vi "DisplayStriptestData.vi"(5 "Strip Lengths [cm]":dbl[](array[numeric]), 6 "min scale array":i32[](array[numeric]), 7 "max scale array":i32[](array[numeric]), 8 "# probed":i32, 9 "Display Stats?":bool, 10 "Thresholds:":T1={"Current [nA]"=200.0, "Ccoupl Lo [pF/cm]"=20.0, "Ccoupl Hi [pF/cm]"=33.0, "Rbias Lo [MW]"=1.0, "Rbias Hi [MW]"=2.0}, 11 "Region":i32) -> (0 "Defects":i32[][](graph), 1 "Resistance [MW]":cluster{u32, i32, "Array OUT":dbl[]}(graph), 2 "Capacitance [pF]":cluster{u32, i32, "Array OUT":dbl[]}(graph), 3 "Current [nA]":cluster{u32, i32, "Array OUT":dbl[]}(graph), 4 "Strip Quality Data":T2 {"pass Rate in %" format="%.2f"})   [LabVIEW 2018]
panel:
  out "max scale":i32
  out "min scale":i32
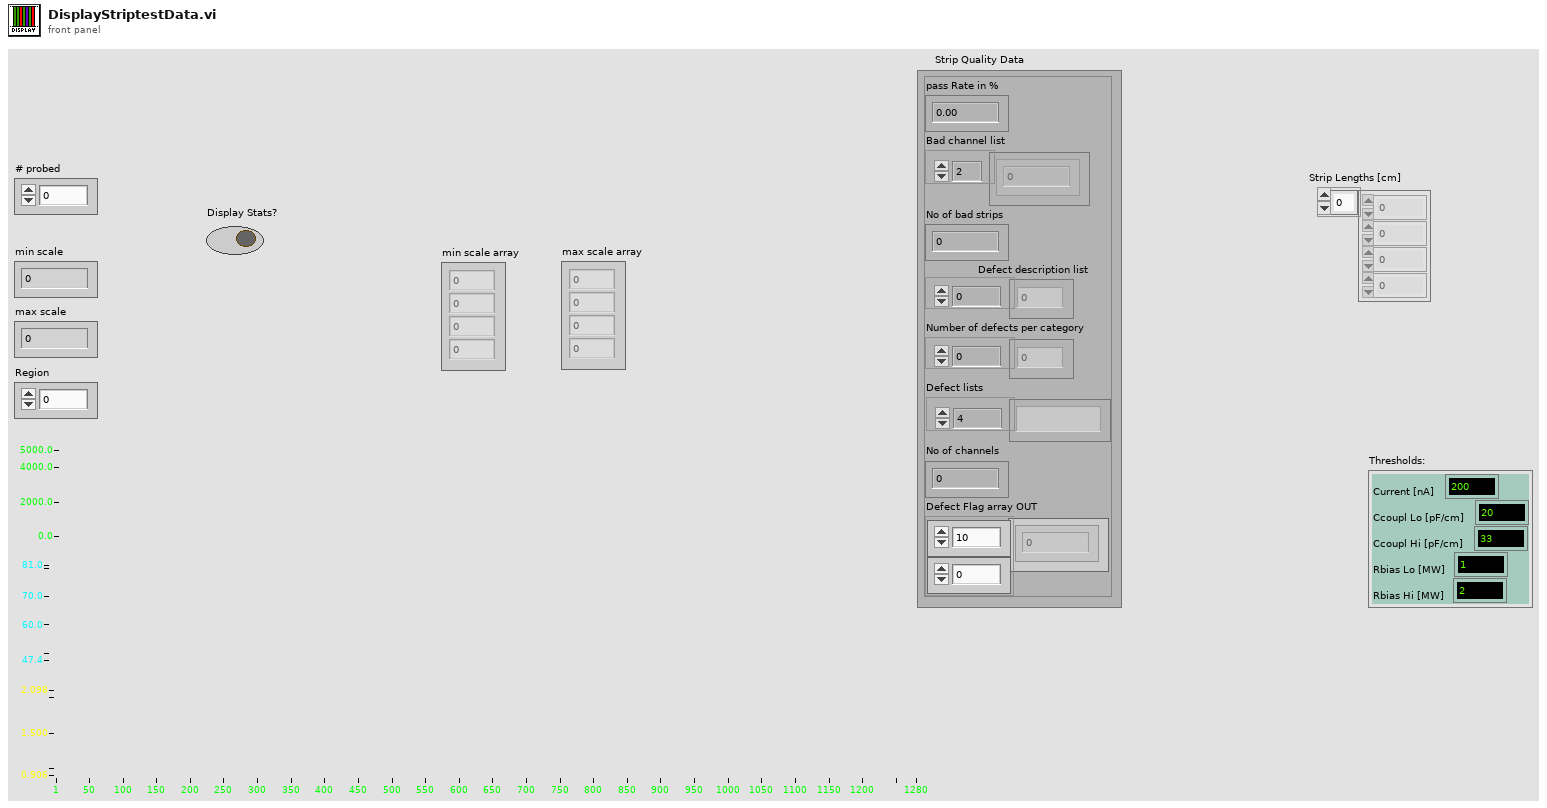
[diagram p1: front panel]
types:
  T1 = cluster{"Current [nA]":dbl, "Ccoupl Lo [pF/cm]":dbl, "Ccoupl Hi [pF/cm]":dbl, "Rbias Lo [MW]":dbl, "Rbias Hi [MW]":dbl}
  T2 = cluster{"pass Rate in %":dbl, "Bad channel list":i32[], "No of bad strips":i32, "Defect description list":i32[], "Number of defects per category":i32[], "Defect lists":string[], "No of channels":i32, "Defect Flag array OUT":i32[][]}
  T3 = enum16{"Reset", "Read Array", "Read Element", "Write Element", "Write Array", "Add Element", "Add Array"}
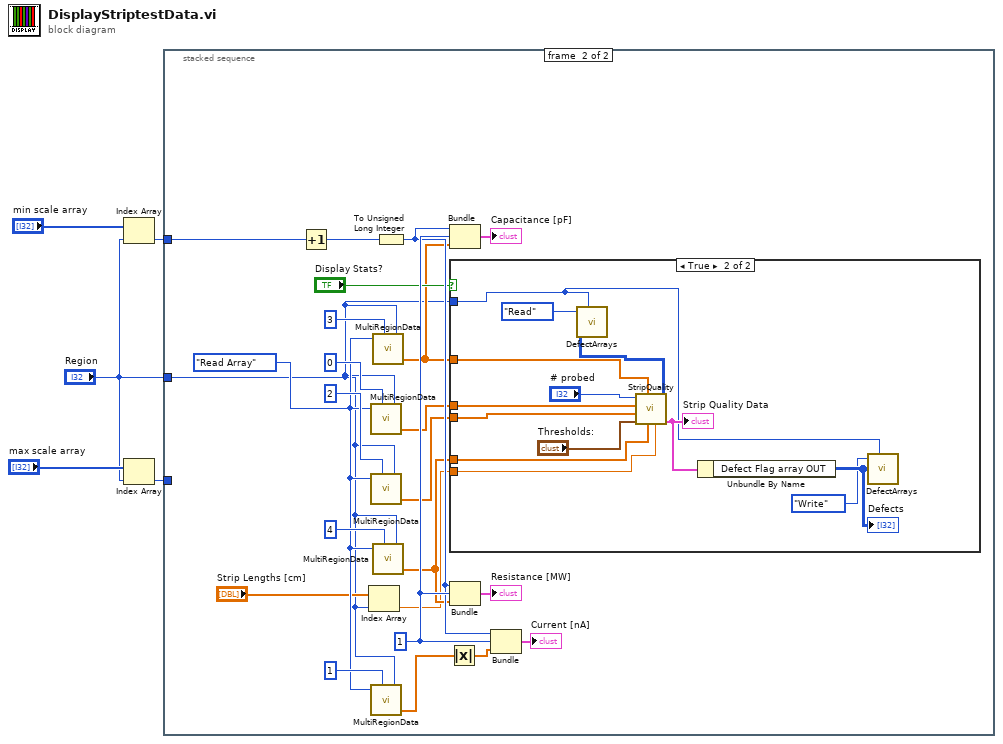
[diagram p0: block diagram]
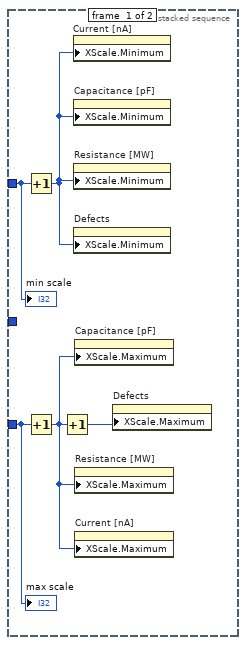
[diagram p2: hidden frame]
diagram:
  n1 = Index Array(array="min scale array", index="Region") -> (element=w4:i32)
  n2 = Index Array(array="max scale array", index="Region") -> (element=w2:i32)
  n3 = stacked-sequence {
    tunnel: w4 -> [w10 w16]
    tunnel: w2 -> [w8 _]
    tunnel: "Region" -> [_ w12]
    frame #0 {
      n4 = Increment(x=w10) -> (x+1=w9:i32)
      n5 = Increment(x=w8) -> (x+1=w7:i32)
      n6 = Increment(x=w7) -> (x+1=w6:i32)
      n7 = property on="Current [nA]" class="WFGraph (strict)"("XScale.Minimum"=w9) -> ()  [unwired: 2 in, 2 out]
      n8 = property on="Capacitance [pF]" class="WFGraph (strict)"("XScale.Minimum"=w9) -> ()  [unwired: 2 in, 2 out]
      n9 = property on="Resistance [MW]" class="WFGraph (strict)"("XScale.Minimum"=w9) -> ()  [unwired: 2 in, 2 out]
      n10 = property on="Defects" class="IntGraph (strict)"("XScale.Minimum"=w9) -> ()  [unwired: 2 in, 2 out]
      n11 = property on="Capacitance [pF]" class="WFGraph (strict)"("XScale.Maximum"=w7) -> ()  [unwired: 2 in, 2 out]
      n12 = property on="Resistance [MW]" class="WFGraph (strict)"("XScale.Maximum"=w7) -> ()  [unwired: 2 in, 2 out]
      n13 = property on="Current [nA]" class="WFGraph (strict)"("XScale.Maximum"=w7) -> ()  [unwired: 2 in, 2 out]
      n14 = property on="Defects" class="IntGraph (strict)"("XScale.Maximum"=w6) -> ()  [unwired: 2 in, 2 out]
      "min scale" <- w10
      "max scale" <- w8
    }
    frame #1 {
      w14 = T3."Read Array" ("Action")
      w28 = 1
      n15 = Increment(x=w16) -> (x+1=w15:i32)
      n16 = Index Array(array="Strip Lengths [cm]", index=w12) -> (element=w11:dbl)
      n17 = call "MultiRegionData.vi"("Action"=w14, "Array No."=0, "Region index"=w12) -> ("Array OUT"=w20:dbl[])  [unwired: 3 in, 1 out]
      n18 = call "MultiRegionData.vi"("Action"=w14, "Array No."=2, "Region index"=w12) -> ("Array OUT"=w17:dbl[])  [unwired: 3 in, 1 out]
      n19 = call "MultiRegionData.vi"("Action"=w14, "Array No."=1, "Region index"=w12) -> ("Array OUT"=w23:dbl[])  [unwired: 3 in, 1 out]
      n20 = call "MultiRegionData.vi"("Action"=w14, "Array No."=3, "Region index"=w12) -> ("Array OUT"=w19:dbl[])  [unwired: 3 in, 1 out]
      n21 = call "MultiRegionData.vi"("Action"=w14, "Array No."=4, "Region index"=w12) -> ("Array OUT"=w18:dbl[])  [unwired: 3 in, 1 out]
      n22 = To Unsigned Long Integer(number=w15) -> (unsigned 32bit integer=w27:u32)
      n23 = Absolute Value(x=w23) -> (abs(x)=w22:dbl[])
      n24 = Bundle(w27, w28, "Array OUT"=w19) -> (→"Capacitance [pF]":cluster{u32, i32, "Array OUT":dbl[]})  [unwired: 1 in]
      n25 = case shown="True" "Display Stats?" {
        tunnel: w20 -> [_ w43]
        tunnel: w19 -> [_ w44]
        tunnel: w18 -> [_ w42]
        tunnel: w17 -> [_ w41]
        tunnel: w12 -> [_ w38]
        tunnel: w11 -> [_ w35]
        frame False {
        }
        frame True {
          n26 = call "DefectArrays.vi"("action"=enum16{"Nothing", "Write", "Read", "Initialise"}."Read", "Region Index"=w38) -> ("Defect array OUT"=w45:i32[][])  [unwired: 1 in, 7 out]
          n27 = call "StripQuality.vi"("Defect Flag array IN"=w45, "Strip Length [cm]"=w35, "Resistance data array"=w42, "Capacitance Data Array"=w44, "Thresholds:"="Thresholds:", "Pinhole flag array in"=w41, "Channel No. Array"=w43, "No of entries"="# probed") -> ("Strip Quality Data"=w40:T2)  [unwired: 2 in, 1 out]
          "Strip Quality Data" <- w40
          n28 = Unbundle By Name(w40) -> ("Defect Flag array OUT"=w39:i32[][])
          "Defects" <- w39
          n29 = call "DefectArrays.vi"("action"=enum16{"Nothing", "Write", "Read", "Initialise"}."Write", "Region Index"=w38, "Defect array IN"=w39) -> ()  [unwired: 8 out]
        }
      }
      n30 = Bundle(w27, w28, "Array OUT"=w18) -> (→"Resistance [MW]":cluster{u32, i32, "Array OUT":dbl[]})  [unwired: 1 in]
      n31 = Bundle(w27, w28, w22) -> (→"Current [nA]":cluster{u32, i32, dbl[]})  [unwired: 1 in]
    }
  }
